vi "limitTo254.vi"(11 "params":u8[](array[numeric])) -> (3 "limitedTo254":u8[](array[numeric]))   [LabVIEW 2014]
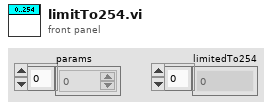
[diagram p1: front panel]
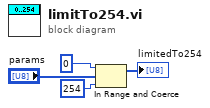
[diagram p0: block diagram]
diagram:
  n1 = In Range and Coerce(upper limit=u8 0, x="params", lower limit=u8 254) -> (coerced(x)=→"limitedTo254":u8[])  [unwired: 1 out]
